vi "Track_T_change_2Ets.vi"(7 "dT Et1":dbl, 10 "T Et 2":dbl, 11 "T Et 1":dbl) -> (2 "T Et 3":dbl, 3 "dT 2":dbl)   [LabVIEW 2010]
panel:
  out "dN/dT interp":dbl[](array[numeric])
  out "DNDT1/DNDT2":dbl
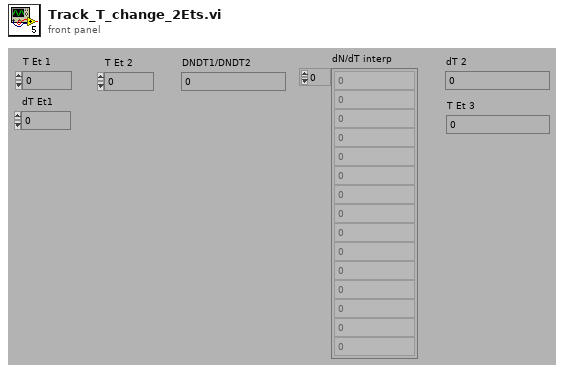
[diagram p1: front panel]
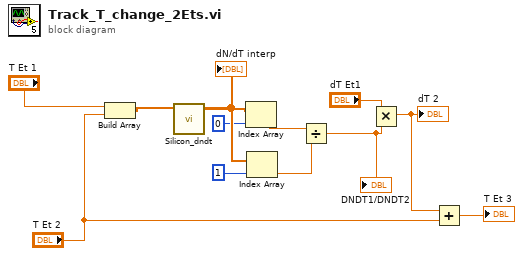
[diagram p0: block diagram]
diagram:
  n1 = Build Array("T Et 1", "T Et 2") -> (w11:dbl[])
  n2 = call "Silicon_dndt.vi"("Temperature"=w11) -> ("dN/dT interp"=w10:dbl[])  [unwired: 10 in]
  "dN/dT interp" <- w10
  n3 = Index Array(array=w10, index=0) -> (element=w7:dbl)
  n4 = Index Array(array=w10, index=1) -> (element=w6:dbl)
  n5 = Divide(x=w7, y=w6) -> (x/y=w4:dbl)
  "DNDT1/DNDT2" <- w4
  n6 = Multiply(x="dT Et1", y=w4) -> (x*y=w3:dbl)
  "dT 2" <- w3
  n7 = Add(x=w3, y="T Et 2") -> (x+y=→"T Et 3":dbl)
